vi "ExecuteSteadyStateProgram.vi"(8 "error in (no error)":errorcluster, 11 "PacificPowerSource in":refnum<class "PacificPowerSource.lvclass">) -> (0 "error out":errorcluster, 3 "PacificPowerSource out":refnum<class "PacificPowerSource.lvclass">)   [LabVIEW 2018, in "AcPwrPlugins.lvlib" / "PacificPowerSource.lvclass"]
uses:
  PacificPowerSource.lvclass
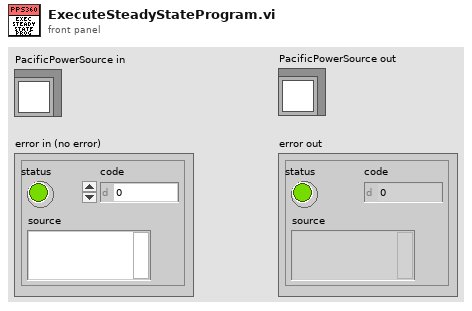
[diagram p1: front panel]
types:
  T1 = typedef "AcPwrPlugins.lvlib/PacificPowerSource.lvclass/LoadSettings.ctl" = cluster{"Handle":string, "Connected":bool, "Impedance Parameters (off, 0.00)":cluster{"State":bool, "Impedance":dbl}, "Source Limits":cluster{"Frequency Minimum (Hz)":dbl, "Frequency Maximum (Hz)":dbl, "Voltage Maximum (V)":dbl, "Voltage Minimum (V)":dbl, "Transition Time (s)":dbl, "Sense":u16, "Set CSC":bool}, "Steady State Parameters":cluster{"Program Name":i32, "Waveform 1":i32, "Waveform 2":i32, "Waveform 3":i32, "Voltage 2":i32, "Voltage 3":i32, "Phase 3":i32, "Current Limit (I)":i32, "Number of Transient Events":i32, "Form":enum16{"Single (1)", "Split (2)", "Three (3)"}, "Coupling":enum16{"Direct", "XFMR"}, "XFMR Ratio":dbl, "Exec Angle":dbl}, "Clear Device":bool, "Configure Output":cluster{"Coupling  (0: Direct)":u16, "Form (3: Three)":u16}, "Range Control (0: Auto)":u16, "Initial Voltage (0V)":u16, "Current Limit (40A)":dbl, "Frequency":cluster{"Frequency High Limit (1200.0Hz)":dbl, "Frequency Low Limit (45Hz)":dbl, "Frequency Range (600Hz)":u16, "Frequency (45Hz)":dbl}, "Waveform":cluster{"Voltage Level (V)":dbl, "Phase (Hz)":i32, "Channel Name (1: A)":u16, "Waveform (1: Sine)":u16}}[]
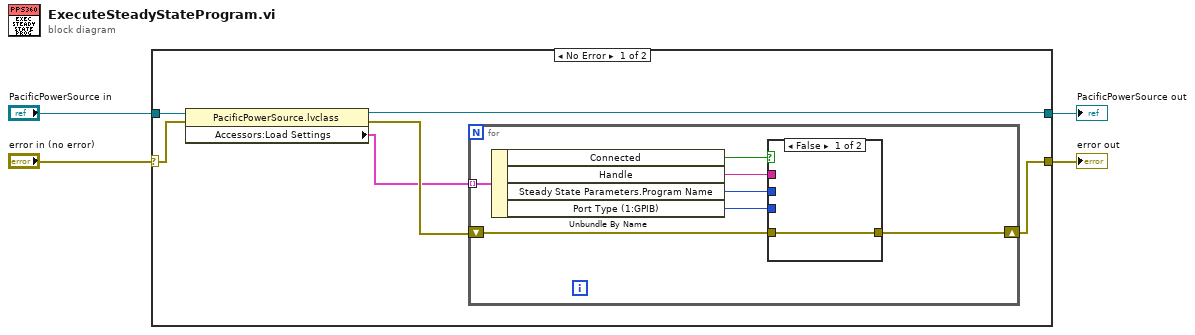
[diagram p0: block diagram]
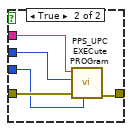
[diagram p2: hidden frame]
diagram:
  n1 = case shown="No Error" "error in (no error)" {
    selector: "error in (no error)" -> [w5 w25]
    tunnel: [w7 w25] -> w4
    tunnel: [w8 w24] -> w3
    tunnel: "PacificPowerSource in" -> [w6 w24]
    frame No Error {
      n2 = property class="PacificPowerSource.lvclass"(reference=w6, error in=w5) -> (reference out=w8:refnum<class "PacificPowerSource.lvclass">, error out=w10:errorcluster, "Accessors:Load Settings"=w9:T1)
      n3 = for {
        tunnel: w9 -> [w17] mode=indexing
        shift-right: [w14] -> w7
        shift-left: w10 -> [w13]
        n4 = Unbundle By Name(w17) -> ("Connected"=w15:bool, "Handle"=w16:string, "Steady State Parameters.Program Name"=w11:i32, "Port Type (1:GPIB)"=w12:enum16{"GPIB", "Serial"})
        n5 = case shown="False" w15 {
          tunnel: w13 -> [w18 w23]
          tunnel: [w18 w22] -> w14
          tunnel: w16 -> [_ w20]
          tunnel: w12 -> [_ w21]
          tunnel: w11 -> [_ w19]
          frame False {
          }
          frame True {
            n6 = call <instrlib>:"PPS_UPC EXECute PROGram.vi"("Port Type"=w21, "error in (no error)"=w23, "Program Name (1)"=w19, "VISA session"=w20) -> ("error out"=w22:errorcluster)  [unwired: 6 in, 1 out]
          }
        }
      }
    }
    frame Error {
    }
  }
  "error out" <- w4
  "PacificPowerSource out" <- w3
